vi "ReadWrite.Data.Commit.vi"(8 "error in":errorcluster, 11 "Ref":T1) -> (0 "error out":errorcluster)   [LabVIEW 2023, in "Plugin Data Access Engine.lvlib" / "Plugin Data Access Engine.lvclass"]
uses:
  Plugin Data Access Engine.lvclass
  Types/ReadWrite.DVR.ctl
  Access Type Classes/ReadWrite/ReadWrite.lvclass
  Access Type Classes/ReadWrite/ReadWrite.lvclass/ReadWrite.ctl
  Plugin Data Access Engine.lvclass/Plugin Data Access Engine.ctl
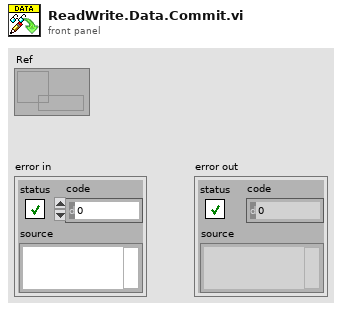
[diagram p1: front panel]
types:
  T1 = typedef "Plugin Data Access Engine.lvlib/Plugin Data Access Engine.lvclass/ReadWrite.DVR.ctl" = refnum<data-value>
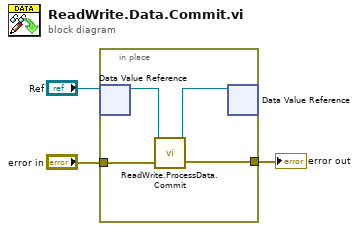
[diagram p0: block diagram]
diagram:
  n1 = in-place {
    in-place-border: "error in" -> [w5]
    in-place-border: [w4] -> w1
    n2 = in-place-dvr #1("Ref") -> (w7:refnum<class "ReadWrite.lvclass">)  [unwired: 1 out]
    n3 = call "ReadWrite.ProcessData.Commit.vi"("error in"=w5, "ReadWrite in"=w7) -> ("error out"=w4:errorcluster, "ReadWrite out"=w6:refnum<class "ReadWrite.lvclass">)  [unwired: 8 in]
    n4 = in-place-dvr #1(w6) -> ()  [unwired: 2 out]
  }
  "error out" <- w1
